vi "RPopLPush.vi"(0 "reference in":refnum<class "Redis.lvclass">, 5 "Source":string, 9 "Destination":string, 11 "Error In":errorcluster) -> (4 "reference out":refnum<class "Redis.lvclass">, 8 "Return":string, 15 "Error Out":errorcluster)   [LabVIEW 2020, in "Redis.lvclass"]
doc: "<b>RPOPLPUSH</b>\n\nAtomically returns and removes the last element (tail) of the list stored at source, and pushes the element at the first element (head) of the list stored at destination.\n\nFor example: consider source holding the list a,b,c, and destination holding the list x,y,z. Executing RPOPLPUSH results in source holding a,b and destination holding c,x,y,z.\n\nIf source does not exist, the value nil is returned and no operation is performed. If source and destination are the same, the operation is equivalent to removing the last element from the list and pushing it as first element of the list, so it can be considered as a list rotation command."
uses:
  Redis.lvclass
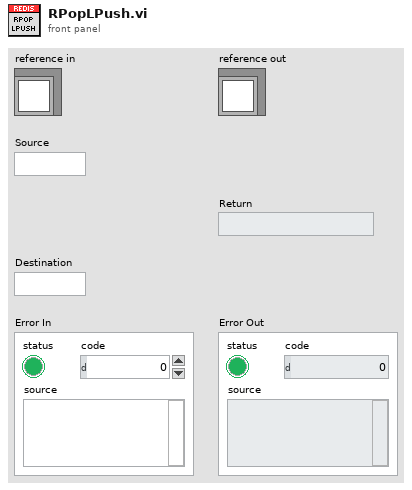
[diagram p1: front panel]
types:
  T1 = typedef "Redis.lvclass/RedisDataType.ctl" = cluster{"Reply Type":T2, "Integer":i64, "String":string, "Multibulk":variant[], "StringData":string[]}
  T2 = typedef "Redis.lvclass/ReplyDataTypeEnum.ctl" = enum16{"None", "Error", "Status", "Nil", "Integer", "String", "Multibulk"}
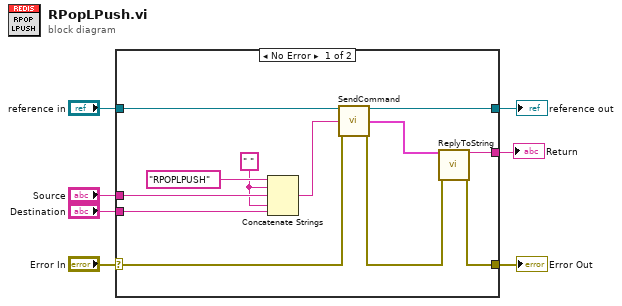
[diagram p0: block diagram]
diagram:
  n1 = case shown="No Error" "Error In" {
    selector: "Error In" -> [w17 w21]
    tunnel: [w8 w21] -> w6
    tunnel: [w19 w20] -> w4
    tunnel: "reference in" -> [w18 w20]
    tunnel: "Source" -> [w15 _]
    tunnel: "Destination" -> [w12 _]
    tunnel: [w10 _] -> w1
    frame No Error {
      w13 = " "
      n2 = Concatenate Strings("RPOPLPUSH", w13, w15, w13, w12) -> (w14:string)
      n3 = call "SendCommand.vi"("reference in"=w18, "Command"=w14, "Error In"=w17) -> ("reference out"=w19:refnum<class "Redis.lvclass">, "Data"=w11:T1, "Error Out"=w9:errorcluster)  [unwired: 10 in]
      n4 = call "ReplyToString.vi"("Reply"=w11, "Error In"=w9) -> ("String"=w10:string, "Error Out"=w8:errorcluster)  [unwired: 12 in]
    }
    frame Error {
    }
  }
  "Error Out" <- w6
  "reference out" <- w4
  "Return" <- w1
